vi "uBroker_Core.vi"(10 "ActorCore Transport":refnum<class "uTransport_uActor.lvclass">, 11 "brokerage queue in":refnum<queue>) -> (3 "brokerage queue out":refnum<queue>)   [LabVIEW 2023, in "uLib.lvlib" / "uBroker.lvclass"]
doc: "This is a helper loop for the actor core. It reduces dynamic dispatching in the brokerage functions as it avoid contiuous recalls of the EXEC method."
uses:
  uBroker.lvclass
  uMsg/uMsg/uMsg.lvclass
  uTransport/uTransport_uActor/uTransport_uActor.lvclass
  TypeDef_uBrokerTopic.ctl
  uClient/uClient_Publisher/uClient_Publisher.lvclass
  U:/Projects/uLib/Src/uFramework/uClient/uClient.lvclass
  uSubscription/uSubscription/uSubscription.lvclass
  uClient/uClient_Subscriber/uClient_Subscriber.lvclass
  uMsg/uMsg/uMsg.lvclass/uMsg.ctl
  uData/uData/uData.lvclass/uData.ctl
  uClient/uClient/uClient.lvclass/uClient.ctl
  uClient/uClient_Subscriber/uClient_Subscriber.lvclass/uClient_Subscriber.ctl
  uPolicy/uPolicy/uPolicy.lvclass/uPolicy.ctl
  uSubscription/uSubscription/uSubscription.lvclass/uSubscription.ctl
  <vilib>/Utility/miscctls.llb/LVMapReplaceAction.ctl
  uClient/uClient_Publisher/uClient_Publisher.lvclass/uClient_Publisher.ctl
  uNotifyMode/uNotifyMode/uNotifyMode.lvclass/uNotifyMode.ctl
  uTransport/uTransport_uActor/uTransport_uActor.lvclass/uTransport_uActor.ctl
  uTransport/uTransport_Event/uTransport_Event.lvclass/uTransport_Event.ctl
  uTransport/uTransport_Queue/uTransport_Queue.lvclass/uTransport_Queue.ctl
  uData/uData/uData.lvclass
  uPolicy/uPolicy/uPolicy.lvclass
  uData/uData/Condition Tag Name.vi
  uClient/uClient/uClient_GetTransport.vi
  uClient/uClient_Subscriber/uSubscriber Get uPolicy.vi
  uPolicy/uPolicy/Read uNotifyMode.vi
  uPolicy/uPolicy/Read uStringManipulation.vi
  uSubscription/uSubscription/uSubscription Update.vi
  uClient/uClient_Publisher/uPublisher GetGUID.vi
  uData/uData/Combine Tags.vi
  uTransport/uTransport/uTransport_SendMsg.vi
  uData/uData/Blank Key Reserved String.vi
  uMsg/uMsg/uMsg Rename CMD.vi
  uNotifyMode/uNotifyMode/uNotify Update.vi
  uMsg/uMsg/uMsg Update Timestamp.vi
  uTransport/uTransport_Event/uTransport_Event_SendMsg.vi
  uTransport/uTransport_Queue/uTransport_Queue_SendMsg.vi
  uNotifyMode/uNotifyMode/uNotifyMode.lvclass
  uTransport/uTransport/uTransport.lvclass
  uStringManipulation/uStringManipulation/uStringManipulation.lvclass
  uTransport/uTransport_Event/uTransport_Event.lvclass
  uTransport/uTransport_Queue/uTransport_Queue.lvclass
  uBroker.lvclass/uBroker.ctl
panel:
  in  "Subscribers":set{refnum<class "uClient_Subscriber.lvclass">}(c389)
  in  "Topics":map{string, T1}(c390)
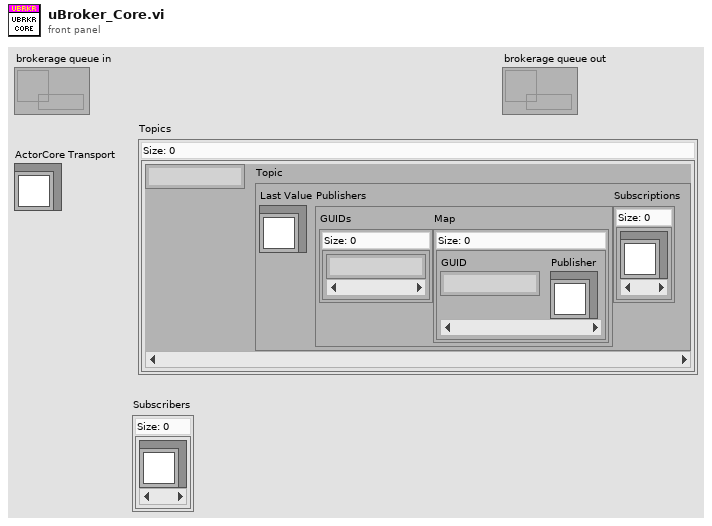
[diagram p1: front panel]
types:
  T1 = typedef "uLib.lvlib/uBroker.lvclass/TypeDef_uBrokerTopic.ctl" = cluster{"Last Value":refnum<class "uMsg.lvclass">, "Publishers":cluster{"GUIDs":set{string}, "Map":map{string, refnum<class "uClient_Publisher.lvclass">}}, "Subscriptions":set{refnum<class "uSubscription.lvclass">}}
  T2 = cluster{"Topics":map{string, T1}, "Subscribers":set{refnum<class "uClient_Subscriber.lvclass">}}
  T3 = typedef "LVMapReplaceAction.ctl" = enum32{"Modify Entry only if found", "Add or Modify Entry", "Delete Entry"}
  T4 = map{string, refnum<class "uClient_Publisher.lvclass">}
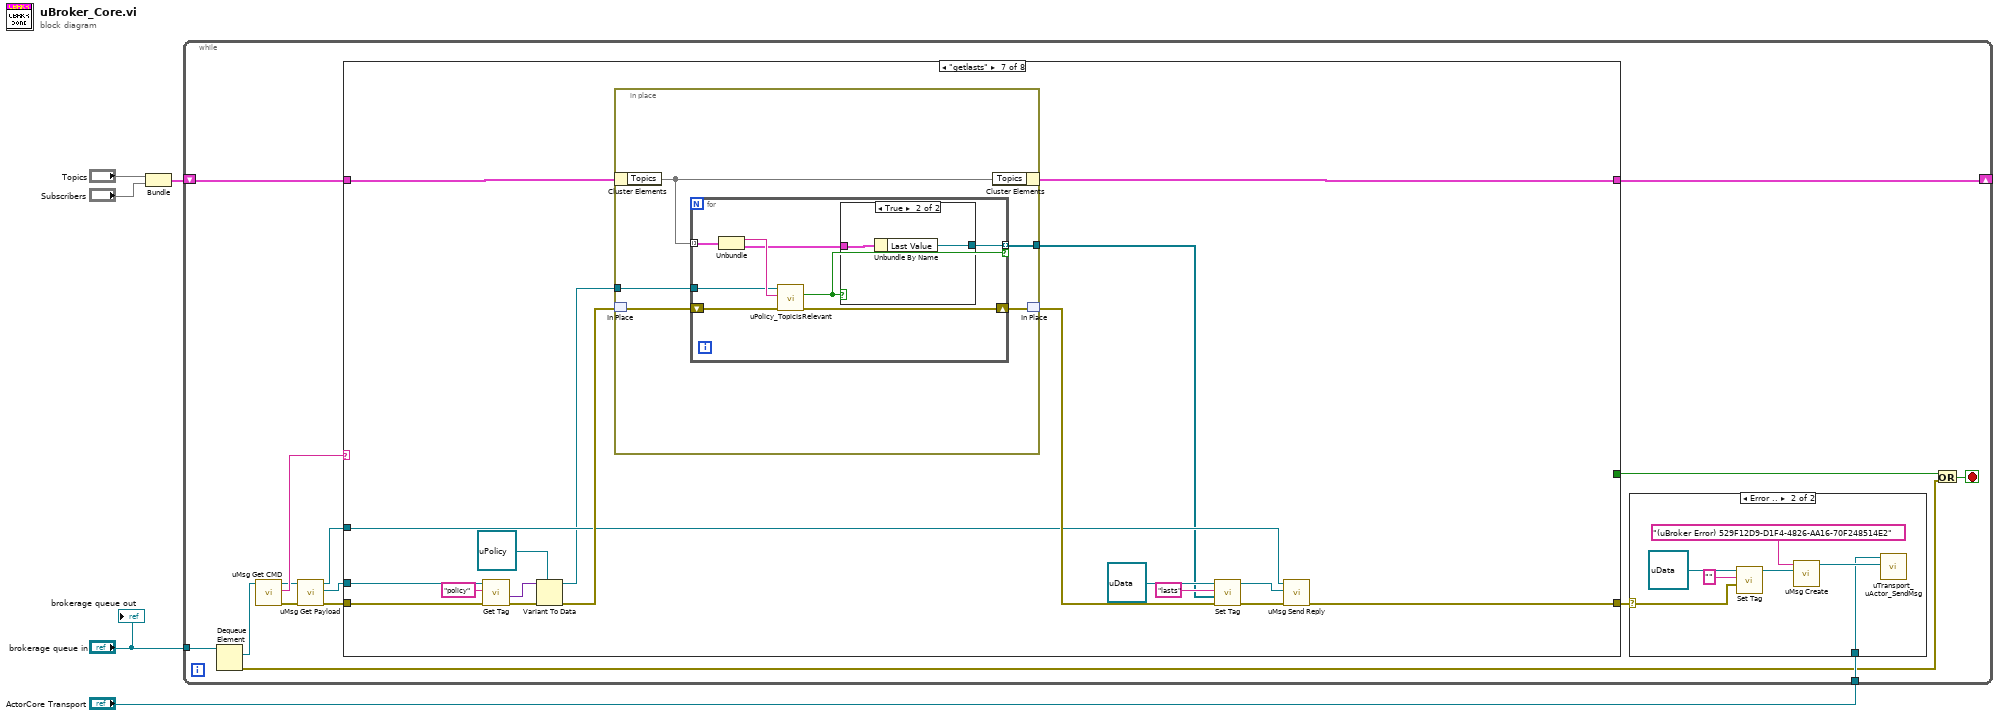
[diagram p0: block diagram]
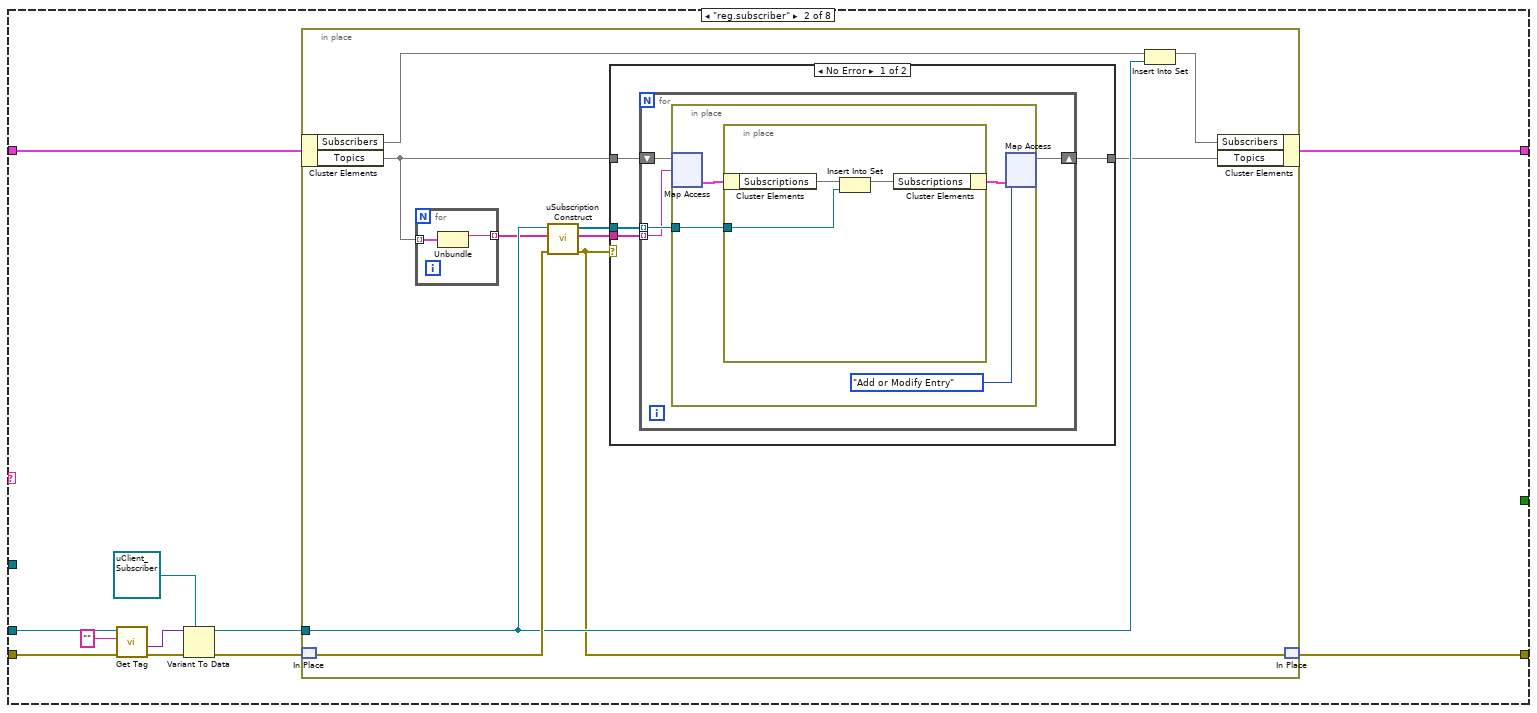
[diagram p4: hidden frame]
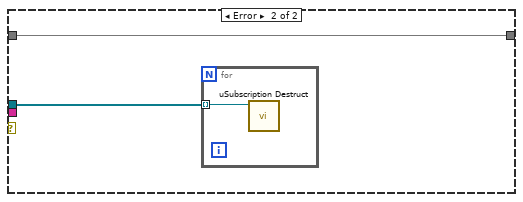
[diagram p5: hidden frame]
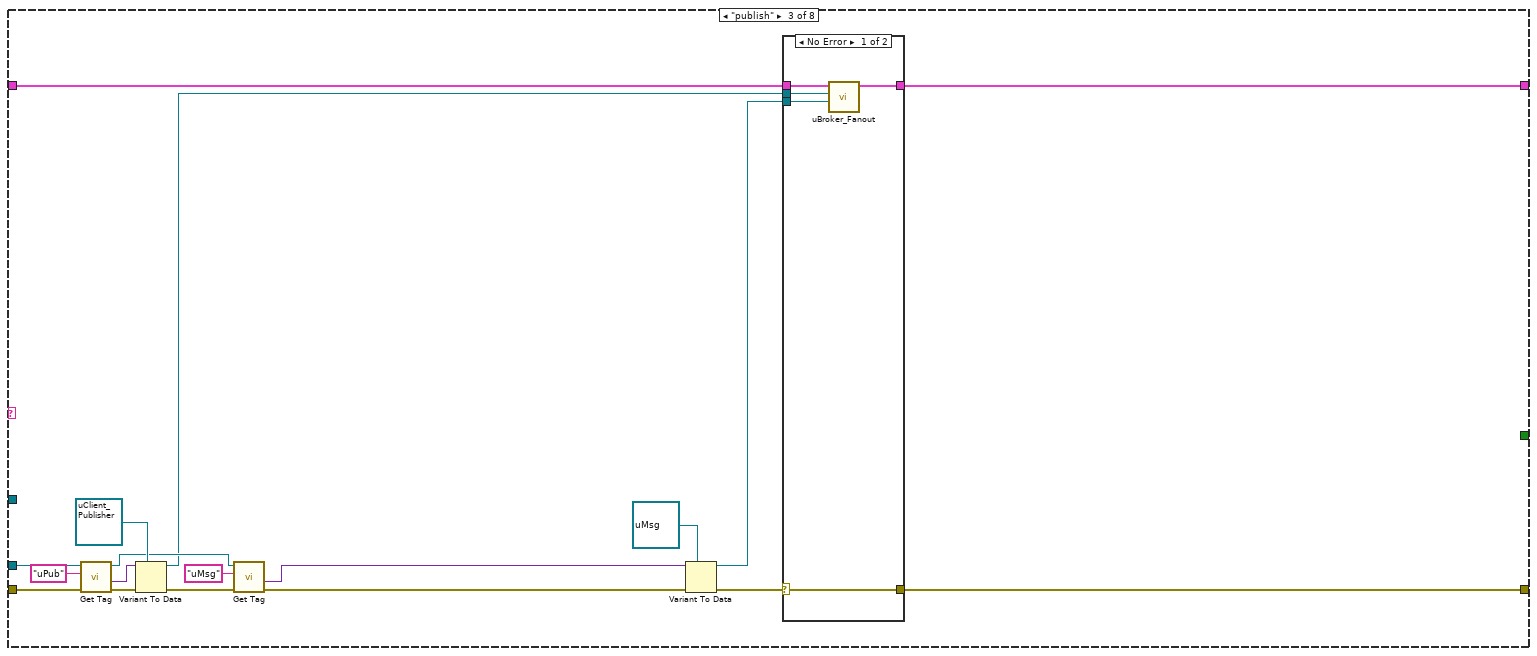
[diagram p6: hidden frame]
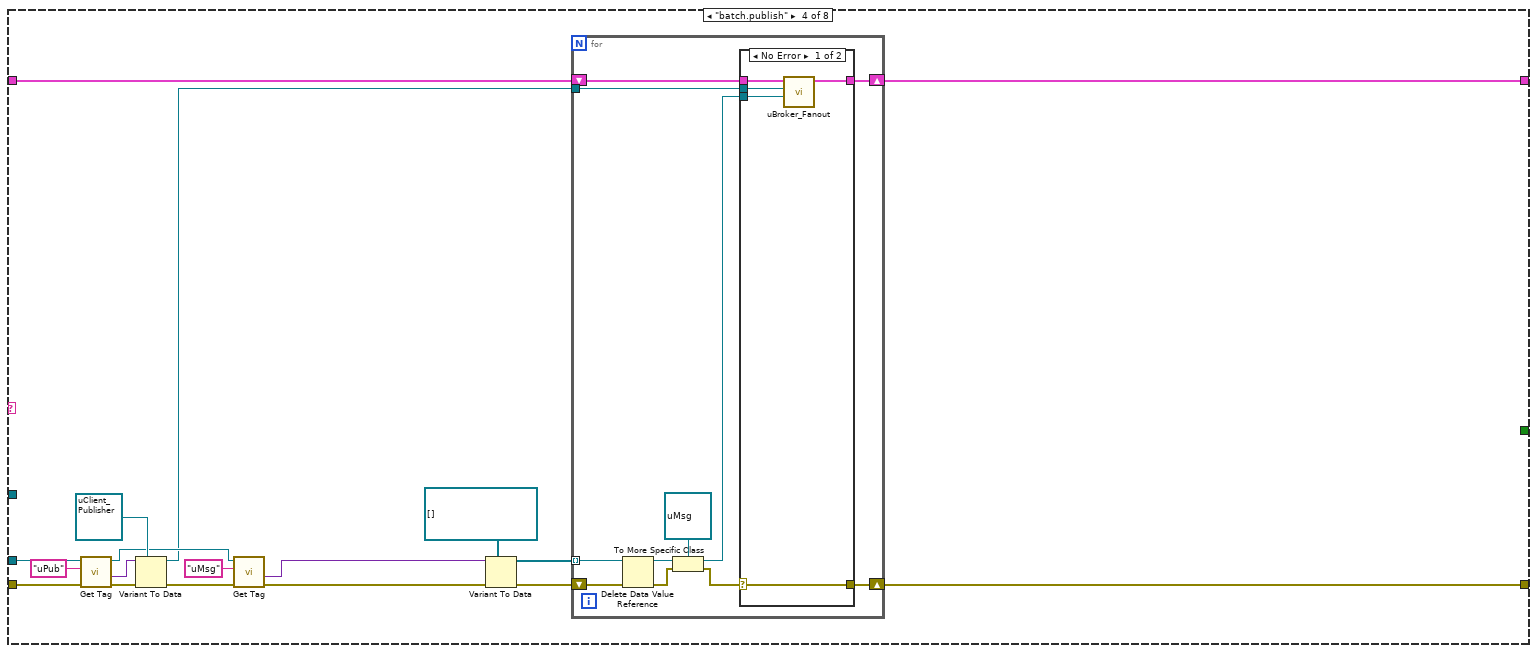
[diagram p8: hidden frame]
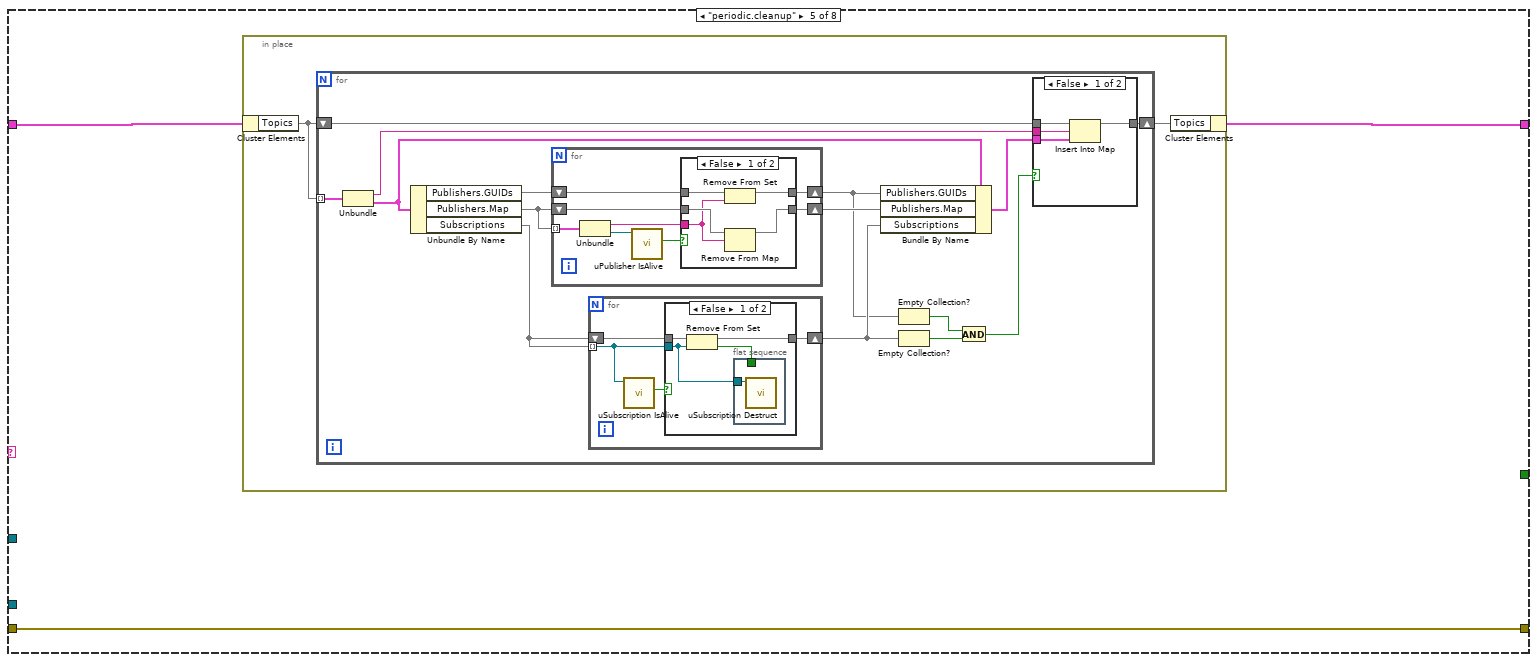
[diagram p10: hidden frame]
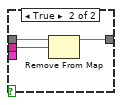
[diagram p11: hidden frame]
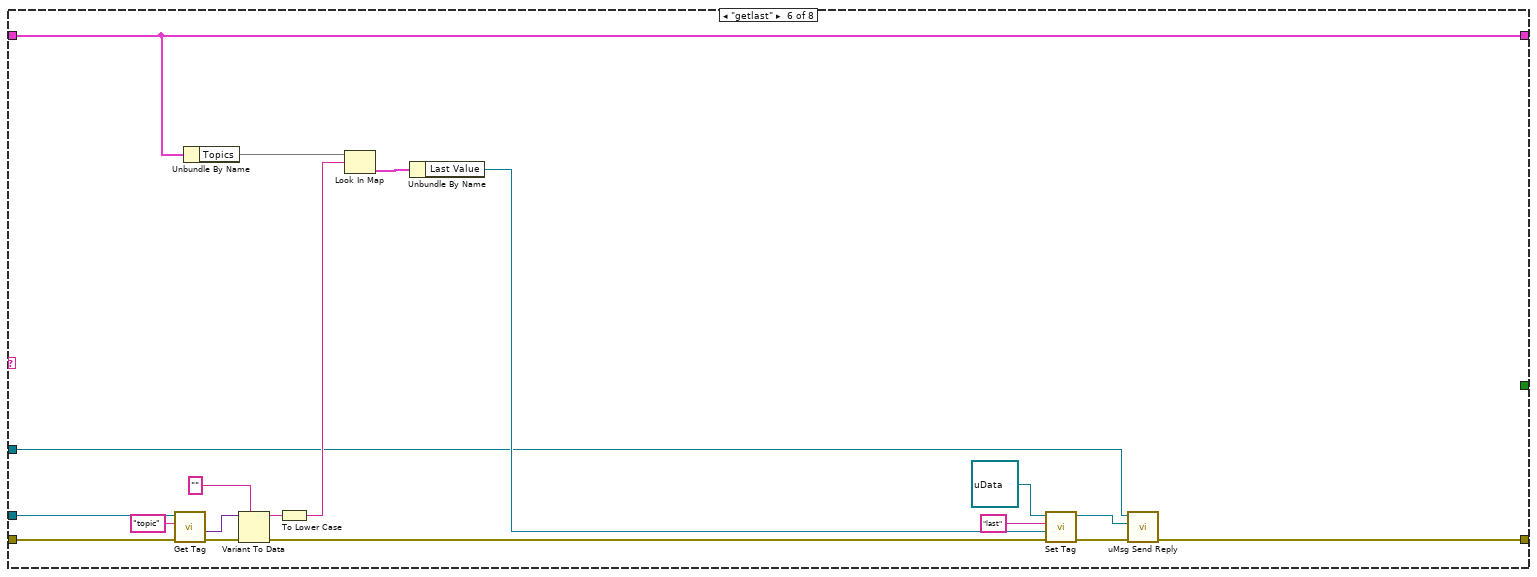
[diagram p14: hidden frame]
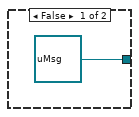
[diagram p15: hidden frame]
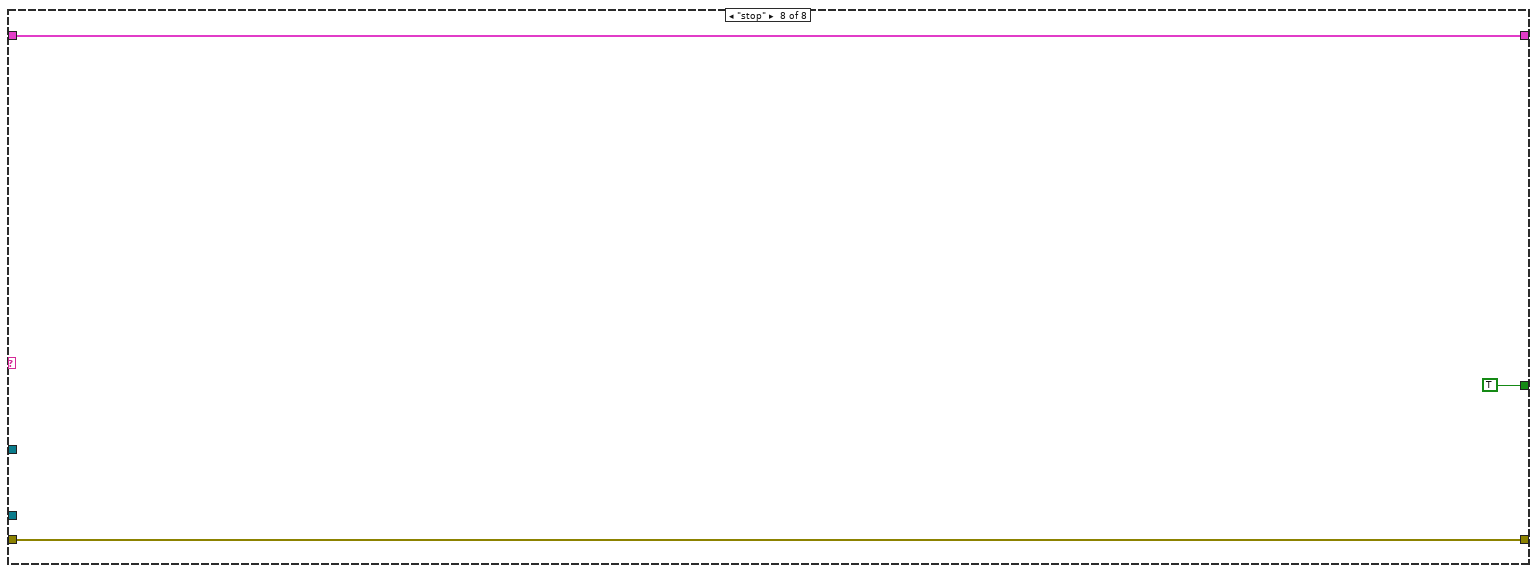
[diagram p16: hidden frame]
diagram:
  n1 = Bundle("Topics"="Topics", "Subscribers"="Subscribers") -> (w3:T2)  [unwired: 1 in]
  n2 = while {
    tunnel: "brokerage queue in" -> [w20]
    tunnel: "ActorCore Transport" -> [w16]
    shift-right: [w14] -> _
    shift-left: w3 -> [w15]
    stop <- w7 stop-if-true
    n3 = Dequeue Element(queue=w20) -> (element=w19:refnum<class "uMsg.lvclass">, error out=w8:errorcluster)  [unwired: 2 in, 2 out]
    n4 = call "uMsg Get CMD.vi"("uMsg in"=w19) -> ("error out"=w13:errorcluster, "CMD"=w18:string, "uMsg out"=w11:refnum<class "uMsg.lvclass">)  [unwired: 8 in]
    n5 = call "uMsg Get Payload.vi"("error in (no error)"=w13, "uMsg in"=w11) -> ("error out"=w12:errorcluster, "uData"=w10:refnum<class "uData.lvclass">, "uMsg out"=w6:refnum<class "uMsg.lvclass">)  [unwired: 7 in]
    n6 = case shown="\"getlasts\"" w18 {
      tunnel: w12 -> [w29 w33 w85 w110 w134 w200 w217 w239]
      tunnel: [w29 w34 w71 w101 w134 w202 w218 w239] -> w17
      tunnel: [w28 w30 w88 w113 w132 w201 w205 w238] -> w14
      tunnel: w15 -> [w28 w31 w87 w112 w133 w201 w206 w238]
      tunnel: w10 -> [_ w32 w86 w111 _ w199 w216 _]
      tunnel: [_ _ _ _ _ _ _ TRUE] -> w9
      tunnel: w6 -> [_ _ _ _ _ w186 w208 _]
      frame Default {
      }
      frame "reg.subscriber" {
        n7 = call "Get Tag.vi"("error in (no error)"=w33, "tag (case insensitive)"="", "uData in"=w32) -> ("error out"=w39:errorcluster, "value"=w38:variant)  [unwired: 5 in, 2 out]
        n8 = Variant To Data(error in=w39, type=refnum<class "uClient_Subscriber.lvclass"> refnum ("uSubscriber"), Variant=w38) -> (data=w36:refnum<class "uClient_Subscriber.lvclass">, error out=w35:errorcluster)
        n9 = in-place {
          in-place-border: w36 -> [w47]
          n10 = in-place-cluster #1(w31) -> ("Subscribers"=w49:set{refnum<class "uClient_Subscriber.lvclass">}, "Topics"=w45:map{string, T1})
          n11 = in-place-match #2(w35) -> (w50:errorcluster)
          n12 = for {
            tunnel: w45 -> [w70] mode=indexing
            tunnel: [w69] -> w46 mode=indexing
            n13 = Unbundle(w70) -> (w69:string)  [unwired: 1 out]
          }
          n14 = call "uSubscription Construct.vi"("error in (no error)"=w50, "Topics"=w46, "uClient_Subscriber"=w47) -> ("error out"=w43:errorcluster, "Filtered Topics"=w41:string[], "uSubscriptions out"=w44:refnum<class "uSubscription.lvclass">[])  [unwired: 6 in]
          n15 = case shown="No Error" w43 {
            tunnel: w45 -> [w54 w67]
            tunnel: w44 -> [w53 w66]
            tunnel: [w52 w67] -> w42
            tunnel: w41 -> [w51 _]
            frame No Error {
              n16 = for {
                tunnel: w53 -> [w57] mode=indexing
                shift-right: [w56] -> w52
                shift-left: w54 -> [w58]
                tunnel: w51 -> [w55] mode=indexing
                n17 = in-place {
                  in-place-border: w57 -> [w59]
                  n18 = in-place-map #3(w58, w55) -> (w61:T1)  [unwired: 1 in, 1 out]
                  n19 = in-place {
                    in-place-border: w59 -> [w63]
                    n20 = in-place-cluster #4(w61) -> ("Subscriptions"=w65:set{refnum<class "uSubscription.lvclass">})
                    n21 = Insert Into Set(10:w63, 11:w65) -> (3:w64:set{refnum<class "uSubscription.lvclass">})  [unwired: 1 out]
                    n22 = in-place-cluster #4("Subscriptions"=w64) -> (w60:T1)
                  }
                  n23 = in-place-map #3(w60, LVMapReplaceAction."Add or Modify Entry" ("action")) -> (w56:map{string, T1})  [unwired: 2 out]
                }
              }
            }
            frame Error {
              n24 = for {
                tunnel: w66 -> [w68] mode=indexing
                n25 = call "uSubscription Destruct.vi"("uSubscription in"=w68) -> ()  [unwired: 10 in, 1 out]
              }
            }
          }
          n26 = Insert Into Set(10:w47, 11:w49) -> (3:w48:set{refnum<class "uClient_Subscriber.lvclass">})  [unwired: 1 out]
          n27 = in-place-cluster #1("Subscribers"=w48, "Topics"=w42) -> (w30:T2)
          n28 = in-place-match #2(w43) -> (w34:errorcluster)
        }
      }
      frame "publish" {
        n29 = call "Get Tag.vi"("error in (no error)"=w85, "tag (case insensitive)"="uPub" ("uPublisher Tag"), "uData in"=w86) -> ("error out"=w83:errorcluster, "value"=w75:variant, "uData out"=w79:refnum<class "uData.lvclass">)  [unwired: 5 in, 1 out]
        n30 = Variant To Data(error in=w83, type=refnum<class "uClient_Publisher.lvclass"> refnum, Variant=w75) -> (data=w76:refnum<class "uClient_Publisher.lvclass">, error out=w81:errorcluster)
        n31 = call "Get Tag.vi"("error in (no error)"=w81, "tag (case insensitive)"="uMsg" ("uPublisher Tag"), "uData in"=w79) -> ("error out"=w78:errorcluster, "value"=w77:variant)  [unwired: 5 in, 2 out]
        n32 = Variant To Data(error in=w78, type=refnum<class "uMsg.lvclass"> refnum ("uFramework.lvlib:uMsg.lvclass"), Variant=w77) -> (data=w74:refnum<class "uMsg.lvclass">, error out=w72:errorcluster)
        n33 = case shown="No Error" w72 {
          selector: w72 -> [w89 w95]
          tunnel: [w93 w94] -> w88
          tunnel: w87 -> [w92 w94]
          tunnel: w76 -> [w91 _]
          tunnel: w74 -> [w90 _]
          tunnel: [w89 w95] -> w71
          frame No Error {
            n34 = call "uBroker_Fanout.vi"("uMsg"=w90, "uPub"=w91, "Cluster in"=w92) -> ("Cluster out"=w93:T2)  [unwired: 8 in]
          }
          frame Error {
          }
        }
      }
      frame "batch.publish" {
        n35 = call "Get Tag.vi"("error in (no error)"=w110, "tag (case insensitive)"="uPub" ("uPublisher Tag"), "uData in"=w111) -> ("error out"=w108:errorcluster, "value"=w99:variant, "uData out"=w104:refnum<class "uData.lvclass">)  [unwired: 5 in, 1 out]
        n36 = Variant To Data(error in=w108, type=refnum<class "uClient_Publisher.lvclass"> refnum, Variant=w99) -> (data=w100:refnum<class "uClient_Publisher.lvclass">, error out=w106:errorcluster)
        n37 = call "Get Tag.vi"("error in (no error)"=w106, "tag (case insensitive)"="uMsg" ("uPublisher Tag"), "uData in"=w104) -> ("error out"=w103:errorcluster, "value"=w102:variant)  [unwired: 5 in, 2 out]
        n38 = Variant To Data(error in=w103, type=refnum<data-value>[] [], Variant=w102) -> (data=w97:refnum<data-value>[], error out=w98:errorcluster)
        n39 = for {
          tunnel: w100 -> [w122]
          tunnel: w97 -> [w121] mode=indexing
          shift-right: [w123] -> w113
          shift-left: w112 -> [w124]
          shift-right: [w115] -> w101
          shift-left: w98 -> [w120]
          n40 = Delete Data Value Reference(data value reference=w121, error in=w120) -> (data value=w118:refnum<class>, error out=w116:errorcluster)
          n41 = To More Specific Class(target class=refnum<class "uMsg.lvclass"> refnum ("uFramework.lvlib:uMsg.lvclass"), reference=w118, error in=w116) -> (specific class reference=w117:refnum<class "uMsg.lvclass">, error out=w114:errorcluster)
          n42 = case shown="No Error" w114 {
            selector: w114 -> [w125 w131]
            tunnel: w124 -> [w129 w130]
            tunnel: [w128 w130] -> w123
            tunnel: w122 -> [w127 _]
            tunnel: w117 -> [w126 _]
            tunnel: [w125 w131] -> w115
            frame No Error {
              n43 = call "uBroker_Fanout.vi"("uMsg"=w126, "uPub"=w127, "Cluster in"=w129) -> ("Cluster out"=w128:T2)  [unwired: 8 in]
            }
            frame Error {
            }
          }
        }
      }
      frame "periodic.cleanup" {
        n44 = in-place {
          n45 = in-place-cluster #5(w133) -> ("Topics"=w135:map{string, T1})
          n46 = for {
            tunnel: w135 -> [w149] mode=indexing
            shift-right: [w146] -> w136
            shift-left: w135 -> [w147]
            n47 = Unbundle(w149) -> (w144:string, "Topic"=w148:T1)
            n48 = Unbundle By Name(w148) -> ("Publishers.GUIDs"=w138:set{string}, "Publishers.Map"=w151:T4, "Subscriptions"=w150:set{refnum<class "uSubscription.lvclass">})
            n49 = for {
              tunnel: w151 -> [w171] mode=indexing
              shift-right: [w175] -> w143
              shift-left: w151 -> [w176]
              shift-right: [w173] -> w137
              shift-left: w138 -> [w172]
              n50 = Unbundle(w171) -> ("GUID"=w169:string, "Publisher"=w170:refnum<class "uClient_Publisher.lvclass">)
              n51 = call "uPublisher IsAlive.vi"("uClient_Publisher in"=w170) -> ("Is Alive?"=w174:bool)  [unwired: 8 in, 2 out]
              n52 = case shown="False" w174 {
                tunnel: w176 -> [w181 w182]
                tunnel: [w180 w182] -> w175
                tunnel: [w178 w183] -> w173
                tunnel: w172 -> [w179 w183]
                tunnel: w169 -> [w177 _]
                frame False {
                  n53 = Remove From Set(10:w177, 11:w179) -> (3:w178:set{string})  [unwired: 1 out]
                  n54 = Remove From Map(10:w177, 11:w181) -> (3:w180:T4)  [unwired: 2 out]
                }
                frame True {
                }
              }
            }
            n55 = for {
              tunnel: w150 -> [w159] mode=indexing
              shift-right: [w161] -> w142
              shift-left: w150 -> [w162]
              n56 = call "uSubscription IsAlive.vi"("uSubscription in"=w159) -> ("Is Alive?"=w160:bool)  [unwired: 9 in, 1 out]
              n57 = case shown="False" w160 {
                tunnel: w162 -> [w166 w168]
                tunnel: [w165 w168] -> w161
                tunnel: w159 -> [w164 _]
                frame False {
                  n58 = Remove From Set(10:w164, 11:w166) -> (2:w163:bool, 3:w165:set{refnum<class "uSubscription.lvclass">})
                  n59 = flat-sequence {
                    tunnel: w164 -> [w167]
                    tunnel: w163 -> [_]
                    frame #0 {
                      n60 = call "uSubscription Destruct.vi"("uSubscription in"=w167) -> ()  [unwired: 10 in, 1 out]
                    }
                  }
                }
                frame True {
                }
              }
            }
            n61 = Bundle By Name(cluster=w148, "Publishers.GUIDs"=w137, "Publishers.Map"=w143, "Subscriptions"=w142) -> (w145:T1)
            n62 = Empty Collection?(1:w137) -> (0:w140:bool)
            n63 = Empty Collection?(1:w142) -> (0:w141:bool)
            n64 = And(x=w140, y=w141) -> (x .and. y?=w139:bool)
            n65 = case shown="False" w139 {
              tunnel: w147 -> [w155 w158]
              tunnel: [w154 w157] -> w146
              tunnel: w145 -> [w153 _]
              tunnel: w144 -> [w152 w156]
              frame False {
                n66 = Insert Into Map(map in=w155, key=w152, value=w153) -> (map out=w154:map{string, T1})  [unwired: 2 out]
              }
              frame True {
                n67 = Remove From Map(10:w156, 11:w158) -> (3:w157:map{string, T1})  [unwired: 2 out]
              }
            }
          }
          n68 = in-place-cluster #5("Topics"=w136) -> (w132:T2)
        }
      }
      frame "getlast" {
        n69 = call "Get Tag.vi"("error in (no error)"=w200, "tag (case insensitive)"="topic", "uData in"=w199) -> ("error out"=w197:errorcluster, "value"=w196:variant)  [unwired: 5 in, 2 out]
        n70 = Unbundle By Name(w201) -> ("Topics"=w184:map{string, T1})
        n71 = Variant To Data(error in=w197, type="" ("tag (case insensitive)"), Variant=w196) -> (data=w195:string, error out=w191:errorcluster)
        n72 = To Lower Case(string=w195) -> (all lower case string=w193:string)
        n73 = Look In Map(map=w184, key=w193) -> (value=w192:T1)  [unwired: 1 in, 1 out]
        n74 = Unbundle By Name(w192) -> ("Last Value"=w189:refnum<class "uMsg.lvclass">)
        n75 = call "Set Tag.vi"("error in (no error)"=w191, "Variant"=w189, "tag (case insensitive)"="last", "uData in"=refnum<class "uData.lvclass"> refnum) -> ("error out"=w185:errorcluster, "uData out"=w187:refnum<class "uData.lvclass">)  [unwired: 5 in, 1 out]
        n76 = call "uMsg Send Reply.vi"("error in (no error)"=w185, "Reply Data"=w187, "Original Msg"=w186) -> ("error out"=w202:errorcluster)  [unwired: 8 in]
      }
      frame "getlasts" {
        n77 = call "Get Tag.vi"("error in (no error)"=w217, "tag (case insensitive)"="policy", "uData in"=w216) -> ("error out"=w214:errorcluster, "value"=w213:variant)  [unwired: 5 in, 2 out]
        n78 = Variant To Data(error in=w214, type=refnum<class "uPolicy.lvclass"> refnum ("tag (case insensitive)"), Variant=w213) -> (data=w204:refnum<class "uPolicy.lvclass">, error out=w220:errorcluster)
        n79 = in-place {
          in-place-border: w204 -> [w224]
          in-place-border: [w221] -> w203
          n80 = in-place-cluster #6(w206) -> ("Topics"=w225:map{string, T1})
          n81 = in-place-match #7(w220) -> (w223:errorcluster)
          n82 = for {
            tunnel: w225 -> [w233] mode=indexing
            tunnel: w224 -> [w231]
            shift-right: [w229] -> w222
            shift-left: w223 -> [w230]
            tunnel: [w227] -> w221 mode=indexing if=w226
            n83 = Unbundle(w233) -> (w232:string, "Topic"=w228:T1)
            n84 = call-dynamic "uPolicy_TopicIsRelevant.vi"("error in (no error)"=w230, "Observed Topic (Lower Case)"=w232, "uPolicy_All in"=w231) -> ("error out"=w229:errorcluster, "Relevant?"=w226:bool)  [unwired: 6 in, 1 out]
            n85 = case shown="True" w226 {
              tunnel: w228 -> [_ w236]
              tunnel: [refnum<class "uMsg.lvclass"> refnum ("Last Value") w235] -> w227
              frame False {
              }
              frame True {
                n86 = Unbundle By Name(w236) -> ("Last Value"=w235:refnum<class "uMsg.lvclass">)
              }
            }
          }
          n87 = in-place-cluster #6("Topics"=w225) -> (w205:T2)
          n88 = in-place-match #7(w222) -> (w219:errorcluster)
        }
        n89 = call "Set Tag.vi"("error in (no error)"=w219, "Variant"=w203, "tag (case insensitive)"="lasts", "uData in"=refnum<class "uData.lvclass"> refnum) -> ("error out"=w207:errorcluster, "uData out"=w209:refnum<class "uData.lvclass">)  [unwired: 5 in, 1 out]
        n90 = call "uMsg Send Reply.vi"("error in (no error)"=w207, "Reply Data"=w209, "Original Msg"=w208) -> ("error out"=w218:errorcluster)  [unwired: 8 in]
      }
      frame "stop" {
      }
    }
    n91 = case shown="Error .." w17 {
      selector: w17 -> [_ w24]
      tunnel: w16 -> [_ w21]
      frame No Error {
      }
      frame Error {
        n92 = call "Set Tag.vi"("Variant"=w24, "tag (case insensitive)"="", "uData in"=refnum<class "uData.lvclass"> refnum) -> ("uData out"=w26:refnum<class "uData.lvclass">)  [unwired: 6 in, 2 out]
        n93 = call "uMsg Create.vi"("Payload"=w26, "CMD"="(uBroker Error) 529F12D9-D1F4-4826-AA16-70F248514E2") -> ("uMsg out"=w22:refnum<class "uMsg.lvclass">)  [unwired: 8 in, 1 out]
        n94 = call "uTransport_uActor_SendMsg.vi"("Msg"=w22, "uTransport_uActor in"=w21) -> ()  [unwired: 9 in, 1 out]
      }
    }
    n95 = Or(x=w9, y=w8) -> (x .or. y?=w7:bool)
  }
  "brokerage queue out" <- "brokerage queue in"
